vi "Get Channel Properties.vi"(8 "error in (no error)":errorcluster, 9 "Number of Paired Channels":i32=4, 10 "Number of DUT-Load Channels":i32=8, 11 "device":refnum<k21>="SLSC-12001-0317E1AA-Mod2") -> (0 "error out":errorcluster, 1 "Channel Pair States":cluster{"name":string, "value":i32}[](array[cluster]), 2 "Channel Bus States":cluster{"name":string, "value":i32}[](array[cluster]), 3 "Channel Load States":cluster{"name":string, "value":i32}[](array[cluster]))   [LabVIEW 2017, in "Routing and Faulting System Tests.lvclass"]
uses:
  Routing and Faulting System Tests.lvclass
  <vilib>/SLSC/Initialize Session with Devices.vi
  <vilib>/SLSC/Get Phys Chan Property (I32).vi
  <vilib>/SLSC/Get Device Property (I32).vi
  <vilib>/SLSC/Close Session.vi
  <vilib>/SLSC/SLSC.lvlib
panel:
  out "SET Chxn Properties":cluster{"name":string, "value":i32}[](array[cluster])
  out "SET Chxp Properties":cluster{"name":string, "value":i32}[](array[cluster])
  in  "Number of 2010 channels":i32=8
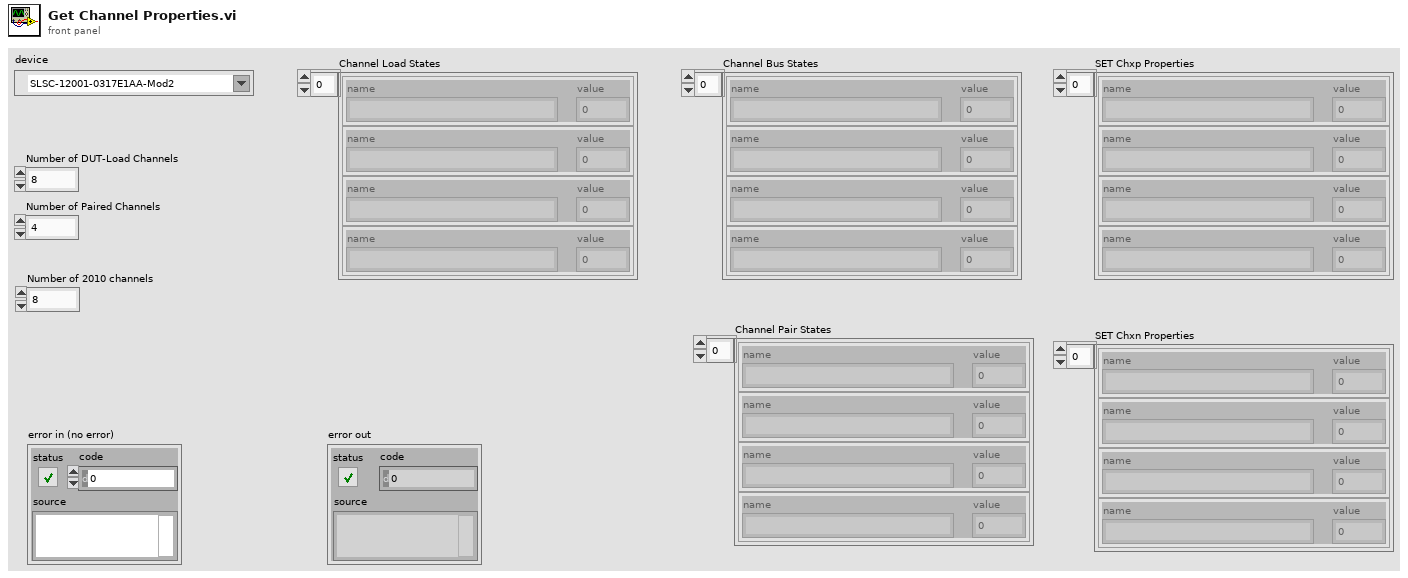
[diagram p1: front panel]
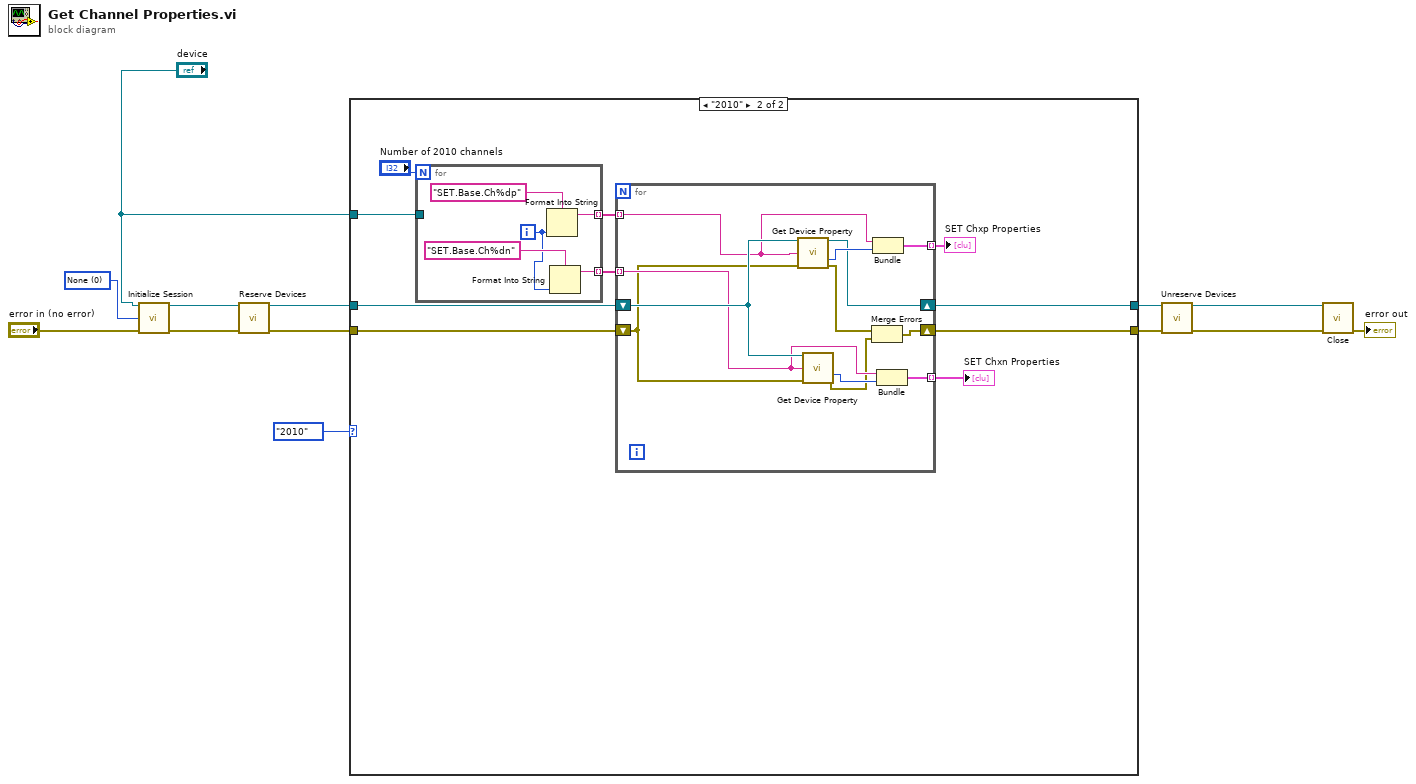
[diagram p0: block diagram]
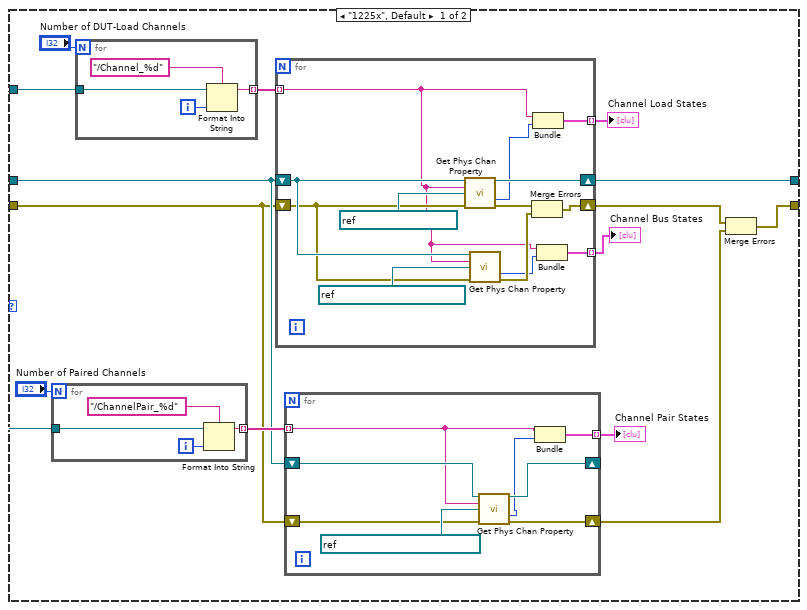
[diagram p2: hidden frame]
diagram:
  w13 = 0 items=["None"=0, "Read Only"=1, "Read/Write"=3] ("reservation access (Read/Write)")
  n1 = call-poly <vilib>:"Initialize Session.vi"("devices"="device", "reservation access (Read/Write)"=w13, "error in (no error)"="error in (no error)") -> ("session out"=w12:refnum<k21>, "error out"=w8:errorcluster)  [unwired: 11 in]
  n2 = call <vilib>:"Reserve Devices.vi"("session in"=w12, "error in (no error)"=w8) -> ("session out"=w5:refnum<k21>, "error out"=w4:errorcluster)  [unwired: 12 in]
  n3 = case shown="\"2010\"" enum16{"1225x", "2010"}."2010" {
    tunnel: [w25 w64] -> w10
    tunnel: w5 -> [w22 w63]
    tunnel: w4 -> [w21 w62]
    tunnel: [w18 w61] -> w3
    tunnel: "device" -> [w14 w60]
    frame "1225x", Default {
      n4 = for {
        N: "Number of Paired Channels" -> [_]
        tunnel: w14 -> [w30]
        tunnel: [w29] -> w23 mode=indexing
        i -> [w28]
        n5 = Format Into String(format string="/ChannelPair_%d", initial string=w30, w28) -> (resulting string=w29:string)  [unwired: 1 in, 1 out]
      }
      n6 = for {
        N: "Number of DUT-Load Channels" -> [_]
        tunnel: w14 -> [w54]
        tunnel: [w55] -> w26 mode=indexing
        i -> [w53]
        n7 = Format Into String(format string="/Channel_%d", initial string=w54, w53) -> (resulting string=w55:string)  [unwired: 1 in, 1 out]
      }
      n8 = for {
        tunnel: w26 -> [w42] mode=indexing
        shift-right: [w51] -> w25
        shift-left: w22 -> [w47]
        shift-right: [w49] -> w19
        shift-left: w21 -> [w46]
        tunnel: [w43] -> w17 mode=indexing
        tunnel: [w40] -> w16 mode=indexing
        n9 = call-poly <vilib>:"Get Phys Chan Property.vi"("session in"=w47, "physical channels"=w42, "property"=refnum<k21> "NI.FIU.State.Load", "error in (no error)"=w46) -> ("session out"=w51:refnum<k21>, "property value"=w44:i32, "error out"=w50:errorcluster)  [unwired: 9 in]
        n10 = call-poly <vilib>:"Get Phys Chan Property.vi"("session in"=w47, "physical channels"=w42, "property"=refnum<k21> "NI.FIU.State.BusSource", "error in (no error)"=w46) -> ("property value"=w41:i32, "error out"=w45:errorcluster)  [unwired: 9 in, 1 out]
        n11 = Merge Errors(w50, w45) -> (w49:errorcluster)
        n12 = Bundle(w42, "property value"=w44) -> (w43:cluster{string, "property value":i32})  [unwired: 1 in]
        n13 = Bundle(w42, "property value"=w41) -> (w40:cluster{string, "property value":i32})  [unwired: 1 in]
      }
      "Channel Load States" <- w17
      "Channel Bus States" <- w16
      n14 = for {
        shift-right: [w35] -> _
        shift-left: w22 -> [w37]
        shift-right: [w36] -> w20
        shift-left: w21 -> [w38]
        tunnel: w23 -> [w34] mode=indexing
        tunnel: [w32] -> w15 mode=indexing
        n15 = call-poly <vilib>:"Get Phys Chan Property.vi"("session in"=w37, "physical channels"=w34, "property"=refnum<k21> "NI.FIU.State.InterChannel", "error in (no error)"=w38) -> ("session out"=w35:refnum<k21>, "property value"=w33:i32, "error out"=w36:errorcluster)  [unwired: 9 in]
        n16 = Bundle(w34, "property value"=w33) -> (w32:cluster{string, "property value":i32})  [unwired: 1 in]
      }
      "Channel Pair States" <- w15
      n17 = Merge Errors(w19, w20) -> (w18:errorcluster)
    }
    frame "2010" {
      n18 = for {
        N: "Number of 2010 channels" -> [_]
        tunnel: w60 -> [_]
        tunnel: [w82] -> w65 mode=indexing
        tunnel: [w79] -> w59 mode=indexing
        i -> [w80]
        n19 = Format Into String(format string="SET.Base.Ch%dp", w80) -> (resulting string=w82:string)  [unwired: 2 in, 1 out]
        n20 = Format Into String(format string="SET.Base.Ch%dn", w80) -> (resulting string=w79:string)  [unwired: 2 in, 1 out]
      }
      n21 = for {
        tunnel: w65 -> [w73] mode=indexing
        shift-right: [w67] -> w64
        shift-left: w63 -> [w74]
        shift-right: [w78] -> w61
        shift-left: w62 -> [w68]
        tunnel: [w77] -> w58 mode=indexing
        tunnel: [w76] -> w57 mode=indexing
        tunnel: w59 -> [w71] mode=indexing
        n22 = call-poly <vilib>:"Get Device Property.vi"("session in"=w74, "property"=w73, "error in (no error)"=w68) -> ("session out"=w67:refnum<k21>, "property value"=w75:i32, "error out"=w70:errorcluster)  [unwired: 10 in]
        n23 = call-poly <vilib>:"Get Device Property.vi"("session in"=w74, "property"=w71, "error in (no error)"=w68) -> ("property value"=w72:i32, "error out"=w69:errorcluster)  [unwired: 10 in, 1 out]
        n24 = Merge Errors(w70, w69) -> (w78:errorcluster)
        n25 = Bundle(w73, "property value"=w75) -> (w77:cluster{string, "property value":i32})  [unwired: 1 in]
        n26 = Bundle(w71, "property value"=w72) -> (w76:cluster{string, "property value":i32})  [unwired: 1 in]
      }
      "SET Chxp Properties" <- w58
      "SET Chxn Properties" <- w57
    }
  }
  n27 = call <vilib>:"Unreserve Devices.vi"("session in"=w10, "error in (no error)"=w3) -> ("session out"=w11:refnum<k21>, "error out"=w7:errorcluster)  [unwired: 12 in]
  n28 = call-poly <vilib>:"Close.vi"("session in"=w11, "error in (no error)"=w7) -> ("error out"=→"error out":errorcluster)  [unwired: 13 in]
